vi "创建设备终端对象.vi"   [LabVIEW 2013, in "个人剂量仪-云服务器.lvclass"]
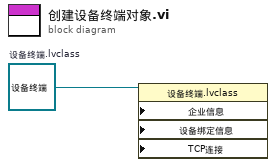
[diagram p0: block diagram]
diagram:
  w1 = refnum<class "设备终端.lvclass"> refnum  # 设备终端.lvclass
  n1 = property class="设备终端.lvclass" props=["企业信息", "设备绑定信息", "TCP连接"](reference=w1) -> ()  [unwired: 4 in, 2 out]
